vi "Read Shutter Status.vi"(8 "error in (no error)":errorcluster, 11 "LTB-1 in":refnum<class "LTB-1.lvclass">) -> (0 "error out":errorcluster, 2 "Shutter Status":bool, 3 "LTB-1 out":refnum<class "LTB-1.lvclass">)   [LabVIEW 2018, in "LTB-1.lvlib" / "LTB-1.lvclass"]
doc: "This VI reads the current attenuation level. It will be overridden by the child class.\n\nThis can be used to confirm the attenuation value is within the specified range.\n\nMAke sure child class returns -1 in error conditions.\n\nAuthor: Ron Dexter\nCompany: Luminar\nModified: 5/20/2018"
uses:
  LTB-1.lvclass
  C:/AME Test Engineering/LabVIEW/PPLs/EXFO/Parent/EXFO.lvlibp/EXFO.lvclass
  LTB-1.lvclass/LTB-1.ctl
  PPLs/EXFO/Parent/EXFO.lvlibp/Methods/Read Resource.vi
  3150 Driver/3150.lvlib
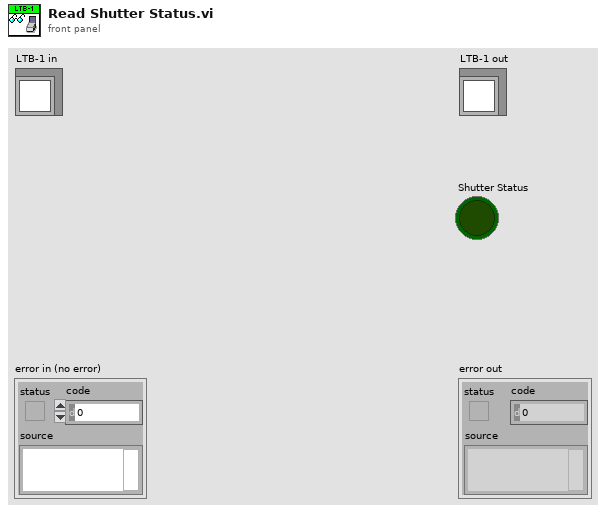
[diagram p1: front panel]
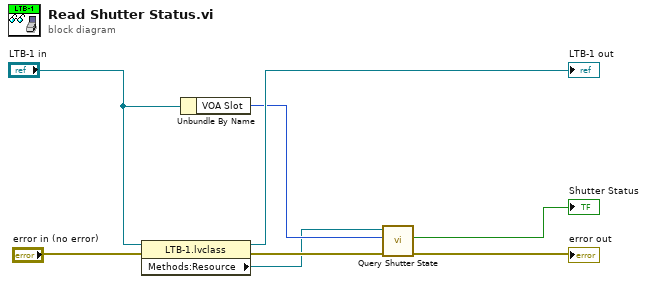
[diagram p0: block diagram]
diagram:
  n1 = property class="LTB-1.lvclass"(reference="LTB-1 in", error in="error in (no error)") -> (reference out=→"LTB-1 out":refnum<class "LTB-1.lvclass">, error out=w5:errorcluster, "Methods:Resource"=w1:refnum<visa-resource-name>)
  n2 = Unbundle By Name("LTB-1 in") -> ("VOA Slot"=w2:i16)
  n3 = call "Query Shutter State.vi"("error in (no error)"=w5, "Platform Slot Number (10)"=w2, "VISA resource name"=w1) -> ("error out"=→"error out":errorcluster, "Shutter State Enabled"=→"Shutter Status":bool)  [unwired: 6 in, 1 out]
